vi "MakeDataFileForVectorplot.vi"(4 "Y Axis Name":string, 6 "X Axis Name":string, 7 "Path":path, 10 "Plot Summary":string[][](array[string]), 11 "XYUVArray":dbl[][](array[numeric])=[[-138.0, 28.0, -5.0, -3.0], [-92.0, 28.0, -10.0, -5.5], [-46.0, 28.0, -5.0, -10.5], [0.0, 28.0, -9.0, 3.5], [46.0, 28.0, -22.0, 1.0], [92.0, 28.0, -24.5, -9.0], [138.0, 28.0, -16.0, -23.0], [-138.0, 60.0, -6.0, -2.0], [-92.0, 60.0, -7.0, -12.0], [-46.0, 60.0, -6.0, -11.0], [0.0, 60.0, -9.0, 3.0], [46.0, 60.0, -5.5, 6.0], [92.0, 60.0, -10.0, -7.5], [138.0, 60.0, -17.0, -22.0], [-138.0, 92.0, 0.5, 2.0], [-92.0, 92.0, -1.5, -15.0], [-46.0, 92.0, -1.5, -10.5], [0.0, 92.0, 1.0, -1.5], [46.0, 92.0, 1.0, 3.0], [92.0, 92.0, -2.5, -7.5], [138.0, 92.0, -5.0, -17.0], [-138.0, 124.0, 18.5, 15.0], [-92.0, 124.0, 10.5, -2.5], [-46.0, 124.0, 6.5, -2.0], [0.0, 124.0, 7.5, 5.0], [46.0, 124.0, 9.5, 12.5], [92.0, 124.0, 14.0, 8.5], [138.0, 124.0, 6.5, -4.0], [-138.0, 156.0, 13.5, 14.5], [-92.0, 156.0, 19.5, 4.0], [-46.0, 156.0, 12.5, -1.0], [0.0, 156.0, 10.5, 3.5], [46.0, 156.0, 14.0, 11.0], [92.0, 156.0, 17.5, 10.5], [138.0, 156.0, 12.0, -4.5], [-138.0, 188.0, 9.0, 16.5], [-92.0, 188.0, 10.0, 8.0], [-46.0, 188.0, 14.0, 4.0], [0.0, 188.0, 15.5, 8.0], [46.0, 188.0, 14.5, 11.0], [92.0, 188.0, 21.5, 11.0], [138.0, 188.0, 19.0, 0.5], [-138.0, 214.0, 12.5, 11.5], [-92.0, 214.0, 17.5, 6.0], [-46.0, 214.0, 17.0, 9.5], [0.0, 214.0, 14.5, 10.5], [46.0, 214.0, 19.0, 10.5], [92.0, 214.0, 20.0, 7.0], [138.0, 214.0, 16.5, 7.0]] caption="X                    Y                      U                  V") -> ()   [LabVIEW 2013]
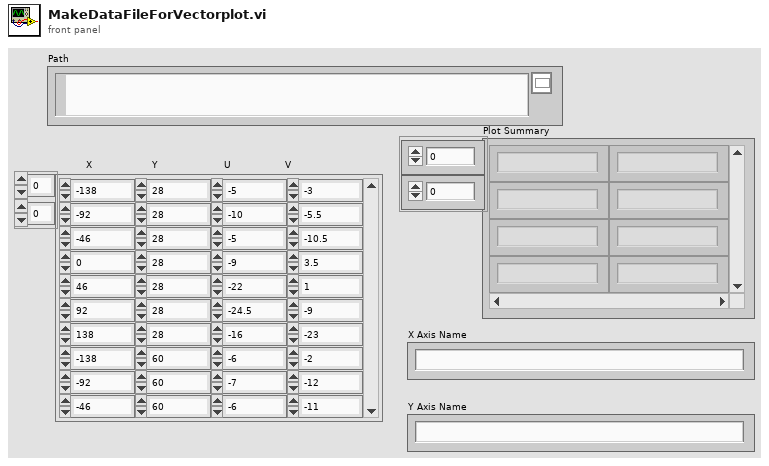
[diagram p1: front panel]
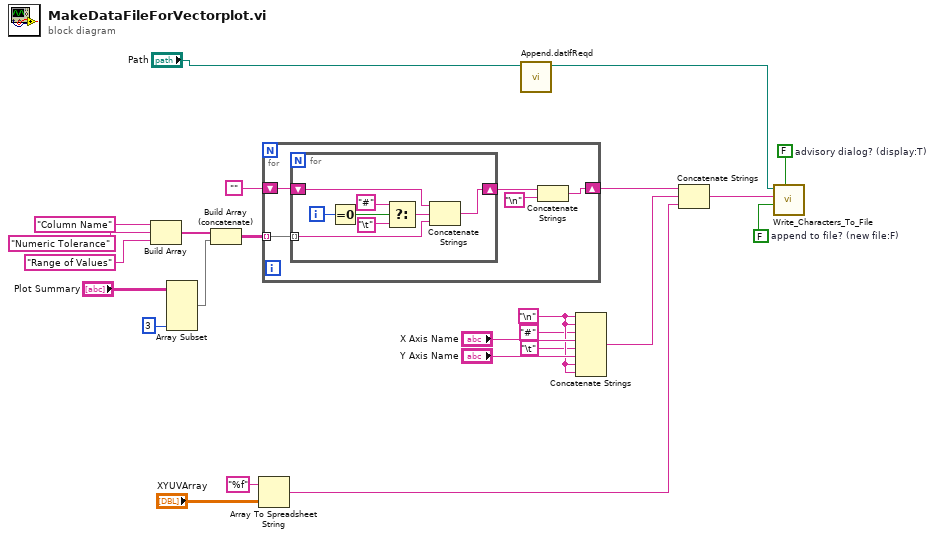
[diagram p0: block diagram]
diagram:
  w9 = FALSE  # advisory dialog? (display:T)
  w8 = FALSE  # append to file? (new file:F)
  w13 = "\n"
  n1 = Build Array("Column Name", "Numeric Tolerance", "Range of Values") -> (w16:string[])
  n2 = Array Subset(array="Plot Summary", length (col)=3 ("length")) -> (w21:string[][])  [unwired: 3 in]
  n3 = Build Array (concatenate)(w16, w21) -> (w23:string[][])
  n4 = Array To Spreadsheet String(array="XYUVArray", 3:"%f" ("format string")) -> (spreadsheet string=w2:string)  [unwired: 1 in]
  n5 = for {
    shift-right: [w28] -> w6
    shift-left: "" -> [w25]
    tunnel: w23 -> [w29] mode=indexing
    n6 = for {
      shift-right: [w30] -> w27
      shift-left: w25 -> [w37]
      tunnel: w29 -> [w31] mode=indexing
      i -> [w36]
      n7 = Equal To 0?(x=w36) -> (x = 0?=w35:bool)
      n8 = Select(t="#", s=w35, f="\t") -> (s? t:f=w32:string)
      n9 = Concatenate Strings(w37, w32, w31) -> (w30:string)
    }
    n10 = Concatenate Strings(w27, "\n") -> (w28:string)
  }
  n11 = call "Append.datIfReqd.vi"("Path"="Path") -> ("appended path"=w10:path)  [unwired: 10 in]
  n12 = Concatenate Strings(w13, w13, "#" ("string"), "X Axis Name", "\t", "Y Axis Name", w13, w13) -> (w5:string)
  n13 = Concatenate Strings(w6, w5, w2) -> (w7:string)
  n14 = call "Write_Characters_To_File.vi"("file path (dialog if empty)"=w10, "advisory dialog? (display:T)"=w9, "character string"=w7, "append to file? (new file:F)"=w8) -> ()  [unwired: 1 in, 4 out]
